vi "CtrlScreenPostion.vi"() -> ()   [LabVIEW 2012]
panel:
  out "error out":errorcluster
  in  "error in (no error)":errorcluster
  in  "Tbl Refnum":refnum<vi>
  # "Not implemented, but block diagram contains some hints about where\nto read the needed properties.\n\nIdea would be to provide a pop-up window with information about the \ncurrent monitor (#, size) of the calling control so that it can position itself\nintellgiently (say at the RHS of the screen)..."
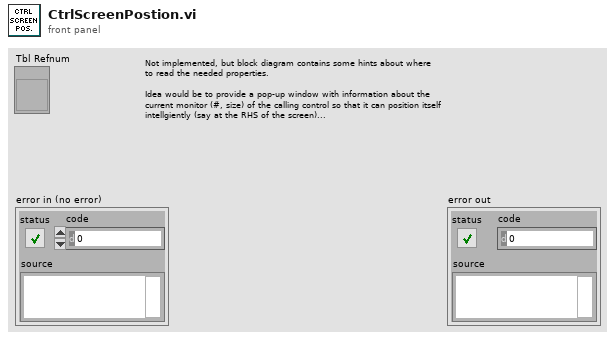
[diagram p1: front panel]
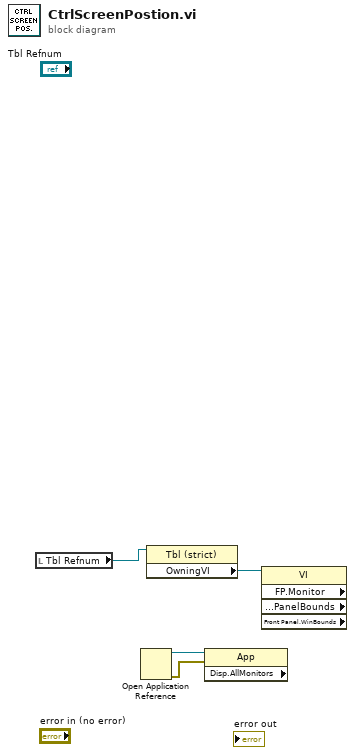
[diagram p0: block diagram]
diagram:
  n1 = local read "Tbl Refnum"() -> (w1:refnum<vi>)
  n2 = Open Application Reference() -> (0:w3:errorcluster, 3:w4:refnum<vi>)  [unwired: 4 in]
  n3 = property class="Tbl (strict)"(reference=w1) -> ("OwningVI"=w2:refnum<vi>)  [unwired: 1 in, 2 out]
  n4 = property class="App" props=["Disp.AllMonitors"](reference=w4, error in=w3) -> ()  [unwired: 3 out]
  n5 = property class="VI" props=["FP.Monitor", "Front Panel.PanelBounds", "Front Panel.WinBounds"](reference=w2) -> ()  [unwired: 1 in, 5 out]
